vi "ep_Check Private Entry Names.vi"(8 "error in (no error)":errorcluster, 11 "entry names":string[](array[string])) -> (0 "error out":errorcluster)   [LabVIEW 2011, in "NI_EP_COMTRADE.lvlib"]
uses:
  <vilib>/addons/Electrical Power/File IO/NI_EP_COMTRADE.lvlib
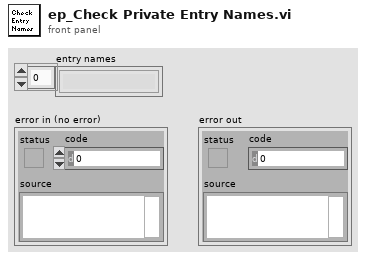
[diagram p1: front panel]
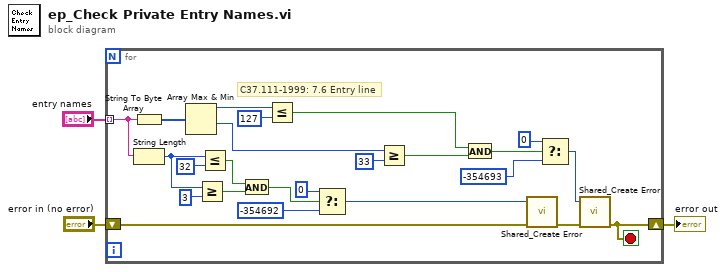
[diagram p0: block diagram]
diagram:
  n1 = for {
    tunnel: "entry names" -> [w23] mode=indexing
    shift-right: [w4] -> w3
    shift-left: "error in (no error)" -> [w9]
    stop <- w4 stop-if-true
    # "C37.111-1999: 7.6 Entry line"
    n2 = String To Byte Array(string=w23) -> (unsigned byte array=w21:u8[])
    n3 = String Length(string=w23) -> (length=w16:i32)
    n4 = Array Max & Min(array=w21) -> (max value=w14:u8, min value=w20:u8)  [unwired: 2 out]
    n5 = Greater Or Equal?(x=w16, y=3) -> (x >= y?=w25:bool)
    n6 = Less Or Equal?(x=w16, y=32 ("x")) -> (x <= y?=w26:bool)
    n7 = And(x=w26, y=w25) -> (x .and. y?=w24:bool)
    n8 = Less Or Equal?(x=w14, y=u8 127 ("x")) -> (x <= y?=w18:bool)
    n9 = Select(t=0 ("error code (0)"), s=w24, f=-354692) -> (s? t:f=w10:i32)
    n10 = Greater Or Equal?(x=w20, y=u8 33) -> (x >= y?=w17:bool)
    n11 = And(x=w18, y=w17) -> (x .and. y?=w19:bool)
    n12 = call <vilib>:"Shared_Create Error.vi"("error in (no error)"=w9, "error code (0)"=w10) -> ("error out"=w8:errorcluster)  [unwired: 9 in]
    n13 = Select(t=0 ("error code (0)"), s=w19, f=-354693 ("error code (0)")) -> (s? t:f=w5:i32)
    n14 = call <vilib>:"Shared_Create Error.vi"("error in (no error)"=w8, "error code (0)"=w5) -> ("error out"=w4:errorcluster)  [unwired: 9 in]
  }
  "error out" <- w3
